vi "ifr2025 RF Type & Units.vi"(8 "error in (no error)":errorcluster {"code" format="%.0x"}, 9 "RF Unit (dBm)":i16(ring) items=["dBm", "dBV", "dBmV", "dBuV", "V", "mV", "uV"], 10 "RF Type (pd)":bool, 11 "instrument handle":refnum<visa-resource-name>) -> (0 "error out":errorcluster {"code" format="%.0x"}, 3 "instrument handle out":refnum<visa-resource-name>)   [LabVIEW 2009]
doc: "This function selects the required units, and EMF or PD for voltage related units."
uses:
  Ifr2025_32.dll
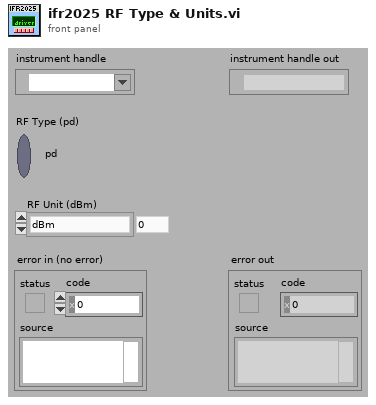
[diagram p1: front panel]
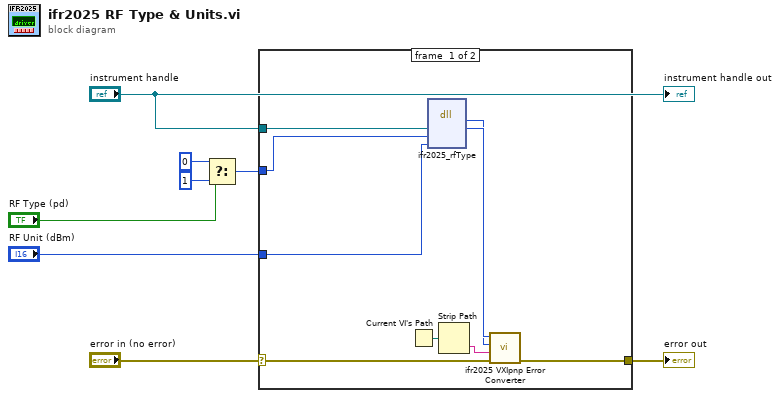
[diagram p0: block diagram]
diagram:
  n1 = Select(t=i16 0, s="RF Type (pd)", f=i16 1) -> (s? t:f=w2:i16)
  n2 = case shown="No Error" "error in (no error)" {
    selector: "error in (no error)" -> [w12 w18]
    tunnel: [w11 w18] -> w8
    tunnel: "instrument handle" -> [w16 _]
    tunnel: w2 -> [w10 _]
    tunnel: "RF Unit (dBm)" -> [w9 _]
    frame #0 {
      n3 = Current VI's Path() -> (path=w17:path)
      n4 = dll-call lib="P:/inst/Marconi 2024 Signal Generator/source/labview/ifr2025/ifr2025/ifr2025_*.*" fn="ifr2025_rfType"("vi"=w16, "RF Type"=w10, "RF Unit"=w9) -> (w14:i32, "vi"=w15:u32)  [unwired: 5 in, 2 out]
      n5 = Strip Path(path=w17) -> (name=w13:string)  [unwired: 1 out]
      n6 = call "ifr2025 VXIpnp Error Converter.vi"("error in (no error)"=w12, "name of VI (\"\")"=w13, "CVI error code (0)"=w14, "instrument handle"=w15) -> ("error out"=w11:errorcluster)  [unwired: 7 out]
    }
    frame #1 {
    }
  }
  "error out" <- w8
  "instrument handle out" <- "instrument handle"
